vi "Post-Bury Template.vi"(6 "Call and Forget?":bool, 8 "Error In":errorcluster, 10 "Grave In":refnum<vi>, 11 "VI In":refnum<vi>) -> (0 "Error Out":errorcluster, 2 "Grave Out":refnum<vi>, 3 "VI Out":refnum<vi>)   [LabVIEW 2018, in "Toolkit.lvlib"]
uses:
  Toolkit.lvlib
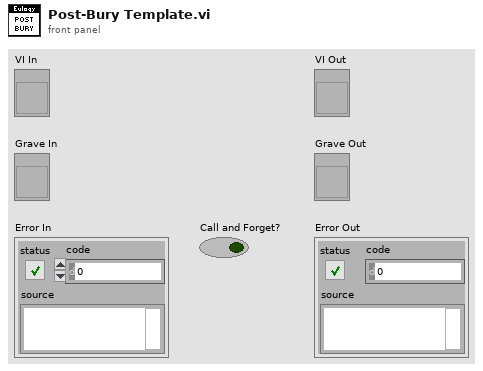
[diagram p1: front panel]
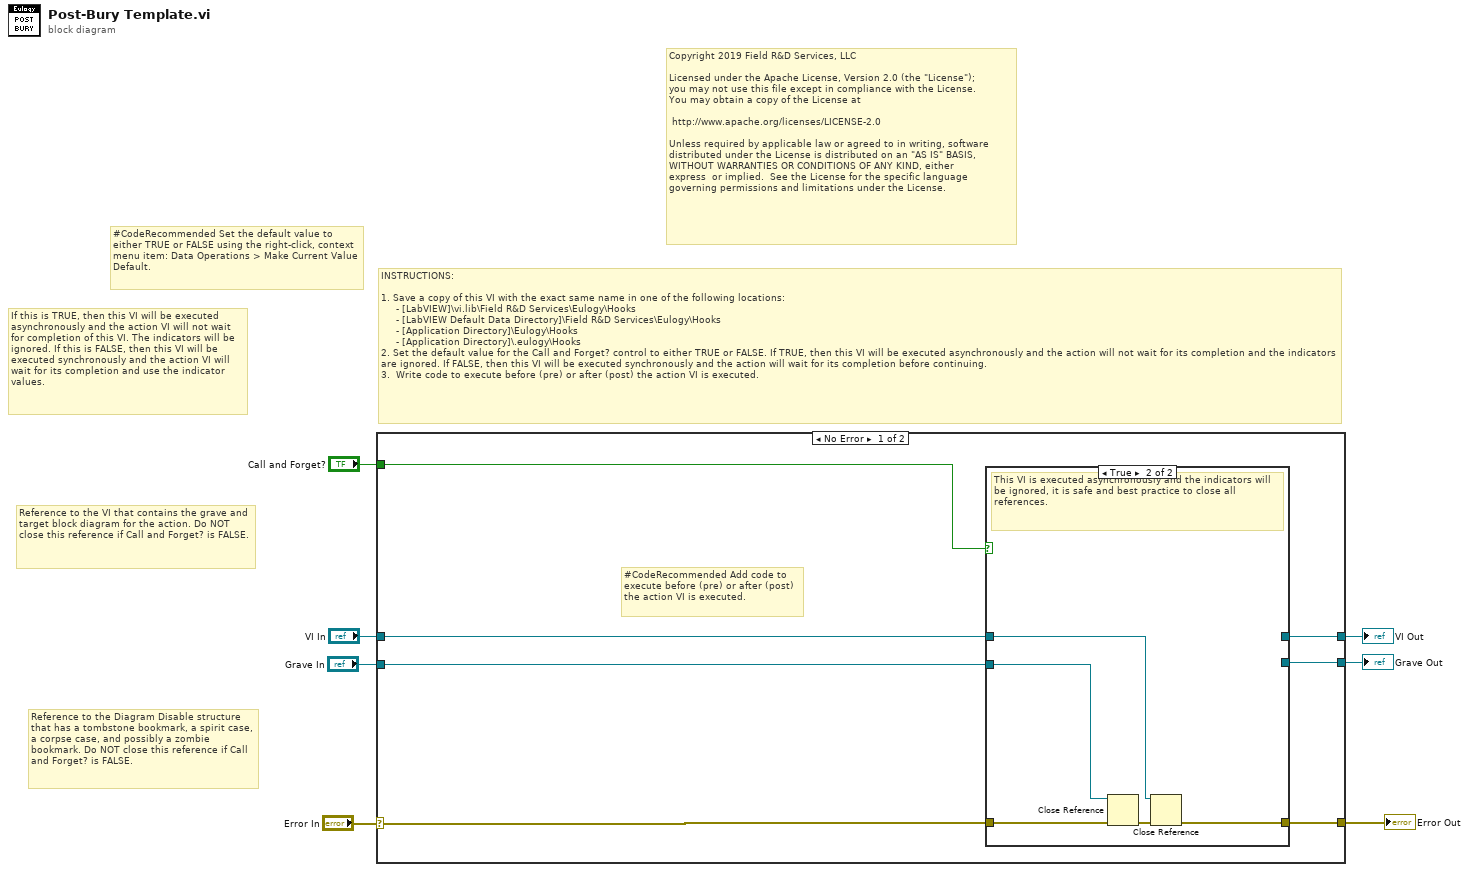
[diagram p0: block diagram]
diagram:
  # "Reference to the Diagram Disable structure that has a tombstone bookmark, a spirit case, a corpse case, and possibly a zombie bookmark. Do NOT close this reference if Call and Forget? is FALSE."
  # "If this is TRUE, then this VI will be executed asynchronously and the action VI will not wait for completion of this VI. The indicators will be ignored. If this is FALSE, then this VI will be executed synchronously and the action VI will wait for its completion and use the indicator values."
  # "Reference to the VI that contains the grave and target block diagram for the action. Do NOT close this reference if Call and Forget? is FALSE."
  # "#CodeRecommended Set the default value to either TRUE or FALSE using the right-click, context menu item: Data Operations > Make Current Value Default."
  # "INSTRUCTIONS:\n\n1. Save a copy of this VI with the exact same name in one of the following locations:\n     - [LabVIEW]\\vi.lib\\Field R&D Services\\Eulogy\\Hooks\n     - [LabVIEW Default Data Directory]\\Field R&D Services\\Eulogy\\Hooks\n     - [Application Directory]\\Eulogy\\Hooks\n     - [Application Directory]\\.eulogy\\Hooks\n2. Set the default value for the Call and Forget? control to either TRUE or FALSE. If TRUE, then this VI will be executed asynchronously and the action will not wait for its completion and the indicators are ignored. If FALSE, then this VI will be executed synchronously and the action will wait for its completion before continuing.\n3.  Write code to execute before (pre) or after (post) the action VI is executed."
  # "Copyright 2019 Field R&D Services, LLC\n\nLicensed under the Apache License, Version 2.0 (the \"License\");\nyou may not use this file except in compliance with the License.\nYou may obtain a copy of the License at\n\n\thttp://www.apache.org/licenses/LICENSE-2.0\n\nUnless required by applicable law or agreed to in writing, software\ndistributed under the License is distributed on an \"AS IS\" BASIS,\nWITHOUT WARRANTIES OR CONDITIONS OF ANY KIND, either \nexpress  or implied.  See the License for the specific language \ngoverning permissions and limitations under the License."
  n1 = case shown="No Error" "Error In" {
    selector: "Error In" -> [w12 w25]
    tunnel: [w11 w25] -> w6
    tunnel: "VI In" -> [w10 w24]
    tunnel: [w8 w24] -> w4
    tunnel: "Call and Forget?" -> [w14 _]
    tunnel: "Grave In" -> [w13 w23]
    tunnel: [w9 w23] -> w1
    frame No Error {
      # "#CodeRecommended Add code to execute before (pre) or after (post) the action VI is executed."
      n2 = case shown="True" w14 {
        tunnel: w13 -> [w17 w22]
        tunnel: w12 -> [w15 w21]
        tunnel: [w15 w19] -> w11
        tunnel: w10 -> [w16 w18]
        tunnel: [w17 _] -> w9
        tunnel: [w16 _] -> w8
        frame False {
          # "This VI is executed synchronously. Do NOT close the references as these will be used by the action VI."
        }
        frame True {
          # "This VI is executed asynchronously and the indicators will be ignored, it is safe and best practice to close all references."
          n3 = Close Reference(reference=w22, error in (no error)=w21) -> (error out=w20:errorcluster)
          n4 = Close Reference(reference=w18, error in (no error)=w20) -> (error out=w19:errorcluster)
        }
      }
    }
    frame Error {
    }
  }
  "Error Out" <- w6
  "Grave Out" <- w1
  "VI Out" <- w4
